vi "onCalculateStatistics.vi"(8 "error in (no error)":errorcluster, 11 "Pips in":refnum<class "Pips.lvclass">) -> (0 "error out":errorcluster, 3 "Pips out":refnum<class "Pips.lvclass">)   [LabVIEW 2021, in "Bananas.lvlib" / "Pips.lvclass"]
uses:
  Pips.lvclass
  pip_filter -- enum.ctl
panel:
  out "% no requirement coverage":dbl
  out "nb non-covered requirements":u32
  out "nb test cases not implemented":u32
  out "nb test cases failed":u32
  out "nb test cases skipped":u32
  out "nb test cases passing":u32
  out "% failed":dbl
  out "nb test cases implemented":u32
  out "% partial requirement coverage":dbl
  out "nb partially covered requirements":u32
  out "% test full coverage":dbl
  out "nb testCases fully covered":u32
  out "nb test cases":u32
  out "% full requirement coverage":dbl
  out "nb fully covered requirements":u32
  out "nb requirements":u32
  out "% pass":dbl
  out "% skipped":dbl
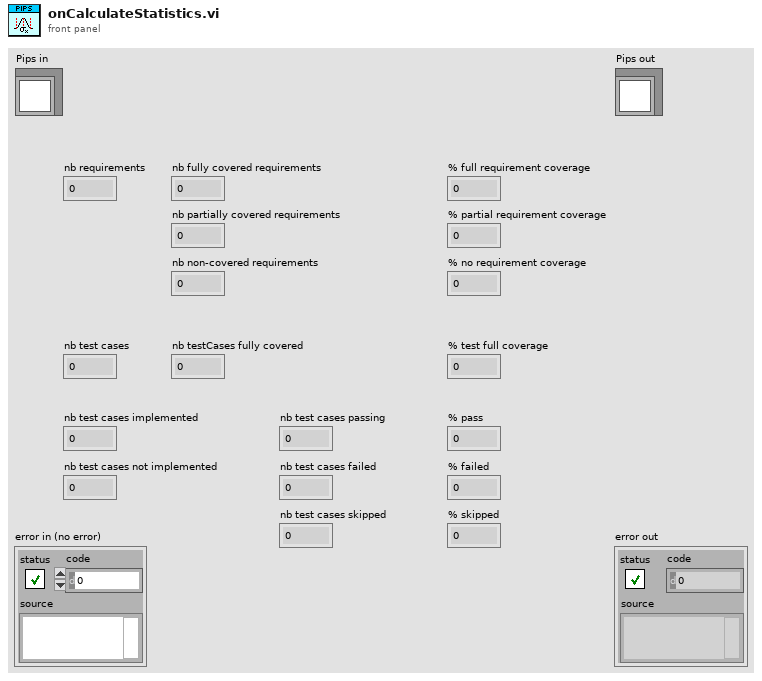
[diagram p1: front panel]
types:
  T1 = typedef "Bananas.lvlib/Pips.lvclass/pip_filter -- enum.ctl" = enum16{"none", "passed", "skipped", "failed", "blocked", "implemented", "covered", "uncovered", "partially-covered"}
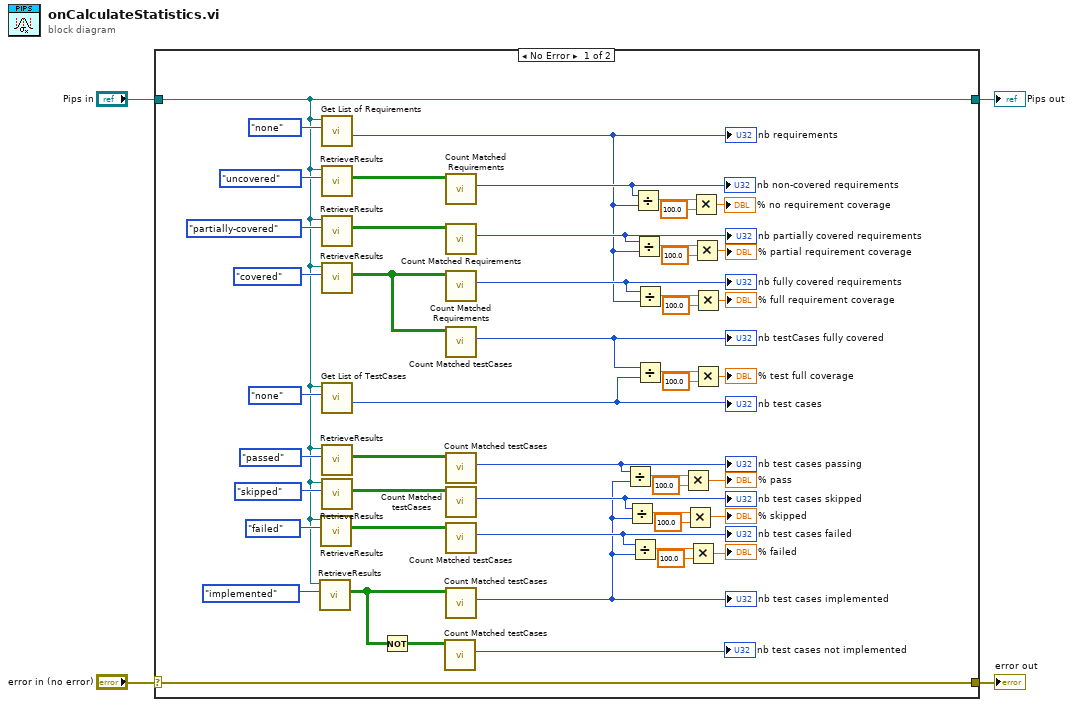
[diagram p0: block diagram]
diagram:
  n1 = case shown="No Error" "error in (no error)" {
    selector: "error in (no error)" -> [w55 w57]
    tunnel: [w55 w57] -> w3
    tunnel: [w10 w56] -> w1
    tunnel: "Pips in" -> [w10 w56]
    frame No Error {
      n2 = call "RetrieveResults.vi"("Filter"=pip_filter_--_enum."implemented", "Pips in"=w10) -> ("Matrix"=w15:bool[][])  [unwired: 7 in, 2 out]
      n3 = call "RetrieveResults.vi"("Filter"=pip_filter_--_enum."failed", "Pips in"=w10) -> ("Matrix"=w26:bool[][])  [unwired: 7 in, 2 out]
      n4 = call "Get List of Requirements.vi"("Filter"=pip_filter_--_enum."none", "Pips in"=w10) -> ("Nb Requirements"=w6:u32)  [unwired: 6 in, 3 out]
      "nb requirements" <- w6
      n5 = call "RetrieveResults.vi"("Filter"=pip_filter_--_enum."uncovered", "Pips in"=w10) -> ("Matrix"=w12:bool[][])  [unwired: 7 in, 2 out]
      n6 = call "RetrieveResults.vi"("Filter"=pip_filter_--_enum."partially-covered", "Pips in"=w10) -> ("Matrix"=w34:bool[][])  [unwired: 7 in, 2 out]
      n7 = call "RetrieveResults.vi"("Filter"=pip_filter_--_enum."covered", "Pips in"=w10) -> ("Matrix"=w32:bool[][])  [unwired: 7 in, 2 out]
      n8 = call "Get List of TestCases.vi"("Filter"=pip_filter_--_enum."none", "Pips in"=w10) -> ("Nb Test Cases"=w35:u32)  [unwired: 6 in, 3 out]
      "nb test cases" <- w35
      n9 = call "RetrieveResults.vi"("Filter"=pip_filter_--_enum."passed", "Pips in"=w10) -> ("Matrix"=w29:bool[][])  [unwired: 7 in, 2 out]
      n10 = call "RetrieveResults.vi"("Filter"=pip_filter_--_enum."skipped", "Pips in"=w10) -> ("Matrix"=w27:bool[][])  [unwired: 7 in, 2 out]
      n11 = Not(x=w15) -> (.not. x?=w14:bool[][])
      n12 = call "Count Matched testCases.vi"("Matrix"=w14) -> ("Nb Test Cases"=→"nb test cases not implemented":u32)  [unwired: 10 in]
      n13 = call "Count Matched Requirements.vi"("Matrix"=w12) -> ("Nb Requirements"=w7:u32)  [unwired: 10 in]
      "nb non-covered requirements" <- w7
      n14 = call "Count Matched Requirements.vi"("Matrix"=w34) -> ("Nb Requirements"=w33:u32)  [unwired: 10 in]
      "nb partially covered requirements" <- w33
      n15 = call "Count Matched Requirements.vi"("Matrix"=w32) -> ("Nb Requirements"=w30:u32)  [unwired: 10 in]
      "nb fully covered requirements" <- w30
      n16 = call "Count Matched testCases.vi"("Matrix"=w32) -> ("Nb Test Cases"=w31:u32)  [unwired: 10 in]
      "nb testCases fully covered" <- w31
      n17 = call "Count Matched testCases.vi"("Matrix"=w29) -> ("Nb Test Cases"=w28:u32)  [unwired: 10 in]
      "nb test cases passing" <- w28
      n18 = call "Count Matched testCases.vi"("Matrix"=w27) -> ("Nb Test Cases"=w23:u32)  [unwired: 10 in]
      "nb test cases skipped" <- w23
      n19 = call "Count Matched testCases.vi"("Matrix"=w26) -> ("Nb Test Cases"=w18:u32)  [unwired: 10 in]
      "nb test cases failed" <- w18
      n20 = call "Count Matched testCases.vi"("Matrix"=w15) -> ("Nb Test Cases"=w17:u32)  [unwired: 10 in]
      "nb test cases implemented" <- w17
      n21 = Divide(x=w28, y=w17) -> (x/y=w24:dbl)
      n22 = Divide(x=w23, y=w17) -> (x/y=w19:dbl)
      n23 = Divide(x=w18, y=w17) -> (x/y=w20:dbl)
      n24 = Divide(x=w7, y=w6) -> (x/y=w9:dbl)
      n25 = Divide(x=w33, y=w6) -> (x/y=w42:dbl)
      n26 = Divide(x=w30, y=w6) -> (x/y=w49:dbl)
      n27 = Divide(x=w31, y=w35) -> (x/y=w45:dbl)
      n28 = Multiply(x=w24, y=100.0) -> (x*y=→"% pass":dbl)
      n29 = Multiply(x=w19, y=100.0) -> (x*y=→"% skipped":dbl)
      n30 = Multiply(x=w20, y=100.0) -> (x*y=→"% failed":dbl)
      n31 = Multiply(x=w9, y=100.0) -> (x*y=→"% no requirement coverage":dbl)
      n32 = Multiply(x=w42, y=100.0) -> (x*y=→"% partial requirement coverage":dbl)
      n33 = Multiply(x=w49, y=100.0) -> (x*y=→"% full requirement coverage":dbl)
      n34 = Multiply(x=w45, y=100.0) -> (x*y=→"% test full coverage":dbl)
    }
    frame Error {
    }
  }
  "error out" <- w3
  "Pips out" <- w1
